vi "FUS-stim.vi"(7 "# Samples in":T1=18000.0 format="%#_9f", 8 "Delay end (ms)":dbl=102.0, 9 "Width of pulse (ms)":dbl=60.0, 11 "Sampling Rate":T1=100000.0 format="%#_9f") -> (0 "Number of Samples (Total)":dbl=28200.0, 1 "Array":dbl[](array[numeric]), 2 "Array 2":T1[](array[typedef]) format="%#_9f", 3 "# Samples out":T1=18000.0 format="%#_9f", 4 "Stimulation 2":cluster{i32, dbl, dbl[]}(graph)={0, 1e-05, array[18000 elements]})   [LabVIEW 2021]
uses:
  Settings.ctl
  <vilib>/measure/NI_MABase.lvlib
panel:
  out "x-y":T1 format="%#_9f"
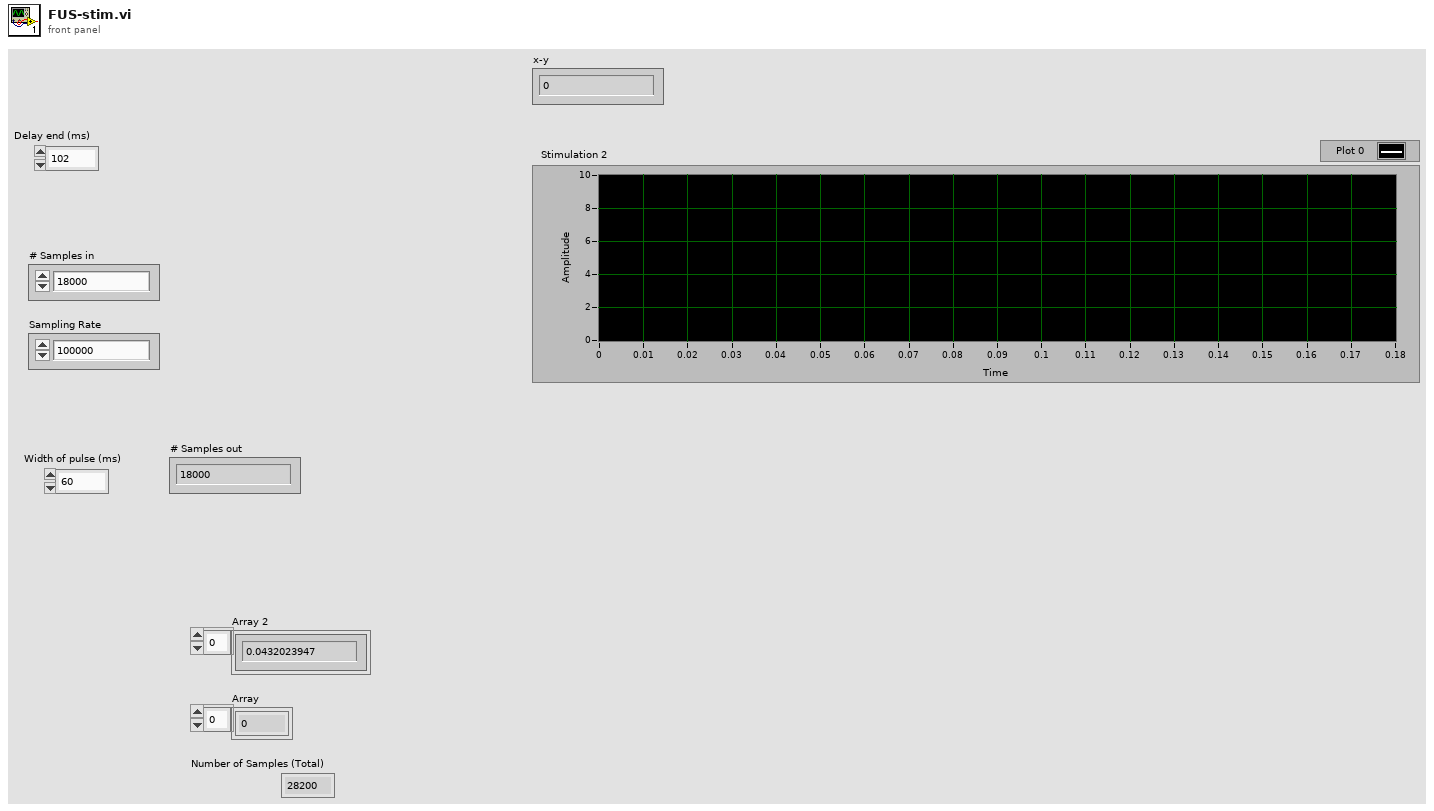
[diagram p1: front panel]
types:
  T1 = typedef "Settings.ctl" = dbl
  T2 = enum16{"Sine Wave", "Triangle Wave", "Square Wave", "Sawtooth Wave"}
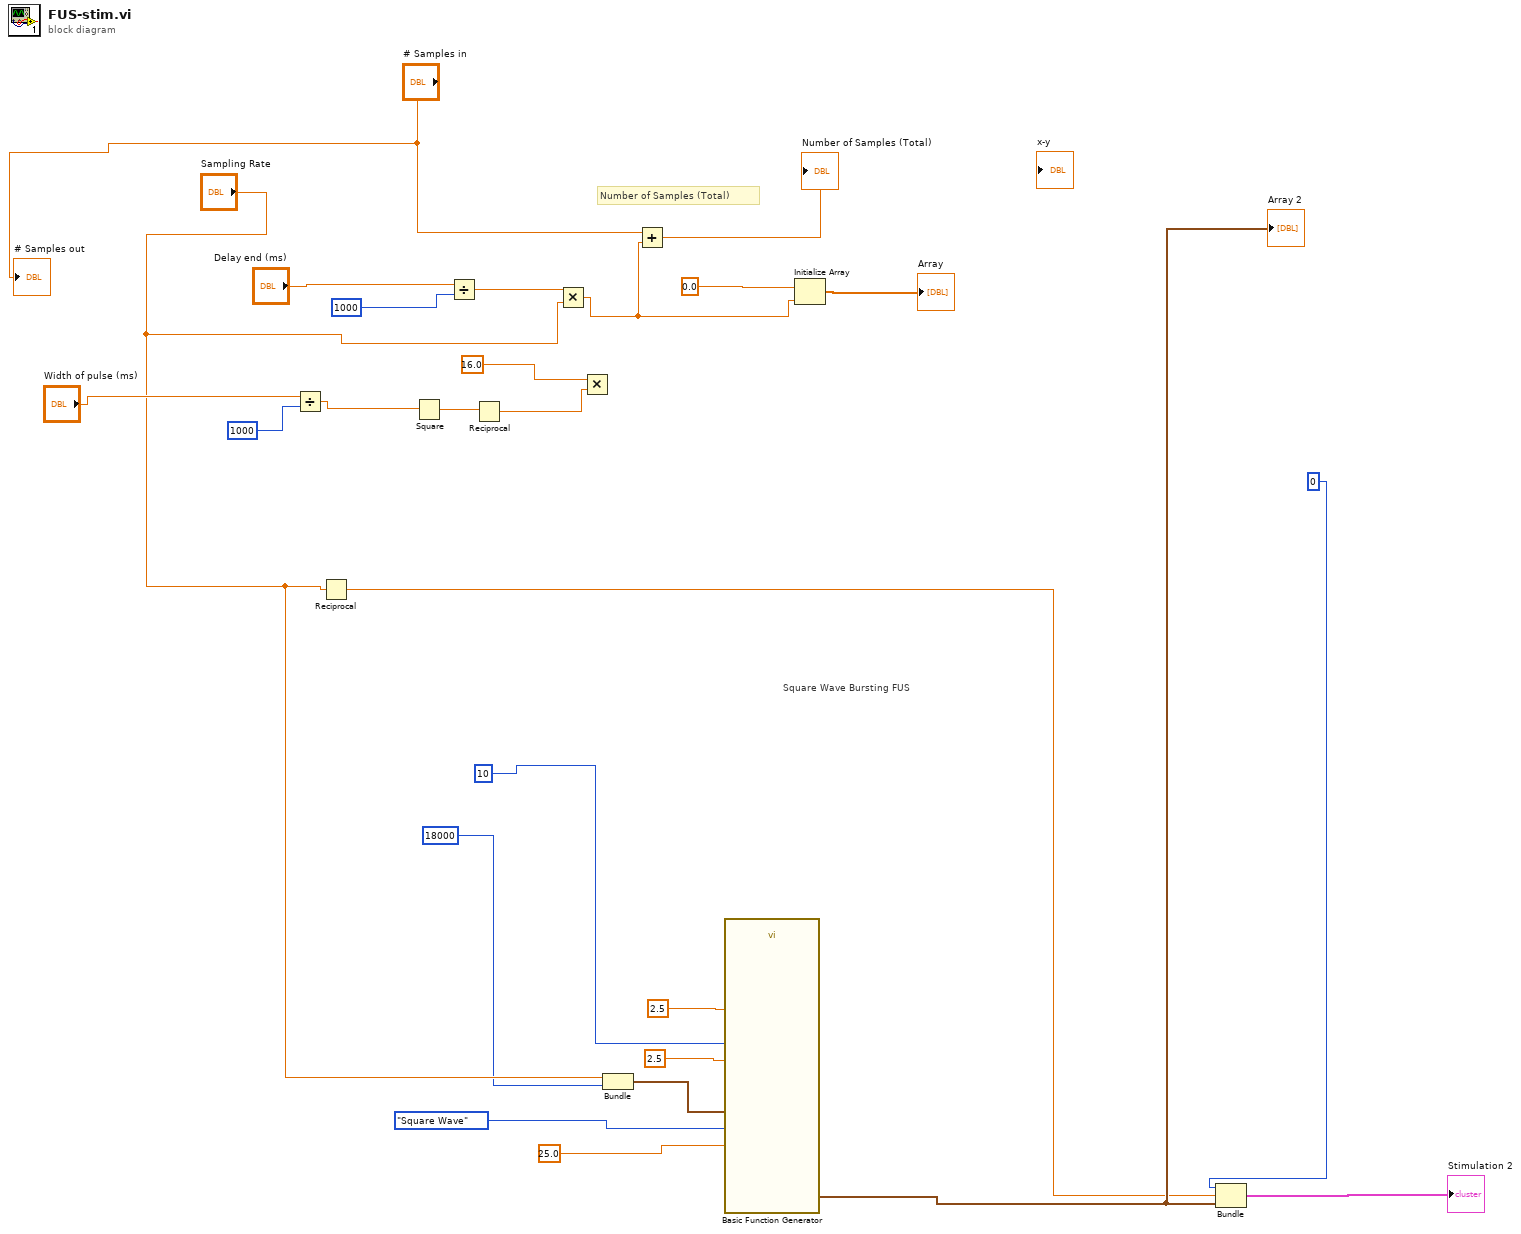
[diagram p0: block diagram]
diagram:
  # "Number of Samples (Total)"
  # "Square Wave Bursting FUS"
  n1 = Divide(x="Width of pulse (ms)", y=1000) -> (x/y=w22:dbl)
  n2 = Reciprocal(x="Sampling Rate") -> (1/x=w2:T1)
  n3 = Square(x=w22) -> (x^2=w18:dbl)
  n4 = Divide(x="Delay end (ms)", y=1000) -> (x/y=w25:dbl)
  n5 = Reciprocal(x=w18) -> (1/x=w19:dbl)
  n6 = Multiply(x=w25, y="Sampling Rate") -> (x*y=w26:T1)
  n7 = Multiply(x=16.0, y=w19) -> ()  [unwired: 1 out]
  n8 = Bundle("Sampling Rate"="Sampling Rate", "samples"=18000) -> (w7:cluster{"Sampling Rate":T1, "samples":i32})  [unwired: 1 in]
  n9 = Add(x="# Samples in", y=w26) -> (x+y=→"Number of Samples (Total)":T1)
  n10 = call <vilib>:"Basic Function Generator.vi"("offset"=2.5, "square wave duty cycle (%)"=25.0, "sampling info"=w7, "signal type"=T2."Square Wave", "amplitude"=2.5, "frequency"=10) -> ("signal out"=w3:waveform(dbl))  [unwired: 3 in, 2 out]
  "Array 2" <- w3
  n11 = Initialize Array(0.0 ("element"), w26) -> (→"Array":dbl[])
  n12 = Bundle(0, w2, "signal out"=w3) -> (→"Stimulation 2":cluster{i32, T1, "signal out":waveform(dbl)})  [unwired: 1 in]
  "# Samples out" <- "# Samples in"
